vi "Read_Status.vi"(8 "error in (no error)":errorcluster, 11 "Modbus master in":refnum<class "Modbus Master.lvclass">) -> (0 "error out":errorcluster, 2 "Variables":u16[](array[numeric]), 3 "Modbus master out":refnum<class "Modbus Master.lvclass">)   [LabVIEW 2019]
uses:
  <vilib>/Modbus/master/Modbus Master.lvclass
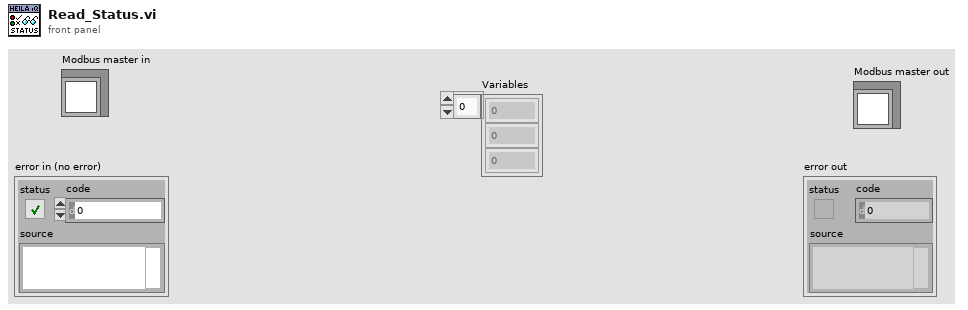
[diagram p1: front panel]
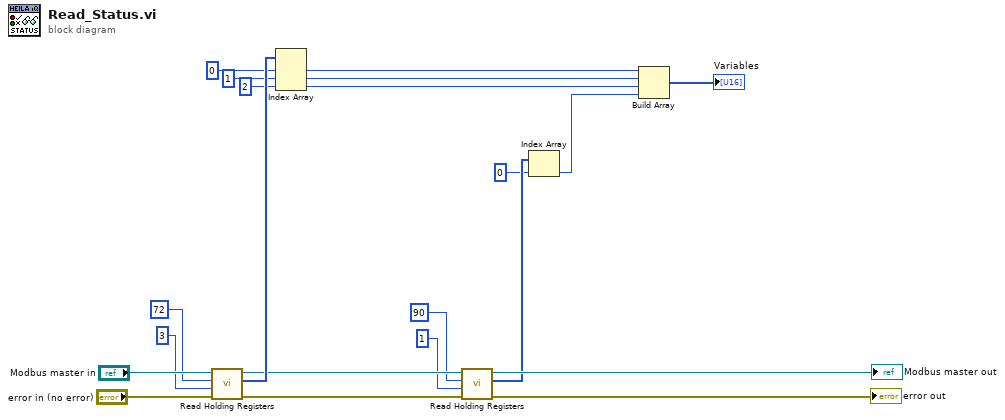
[diagram p0: block diagram]
diagram:
  n1 = call-dynamic "Read Holding Registers.vi"("error in (no error)"="error in (no error)", "number of holding registers"=u16 3 ("starting address"), "starting address"=u16 72, "Modbus master in"="Modbus master in") -> ("error out"=w8:errorcluster, "register values"=w17:u16[], "Modbus master out"=w9:refnum<class "Modbus Master.lvclass">)  [unwired: 5 in]
  n2 = Index Array(array=w17, index #1=0 ("index"), index #2=1 ("index"), index #3=2 ("index")) -> (element #1=w13:u16, element #2=w12:u16, element #3=w11:u16)
  n3 = call-dynamic "Read Holding Registers.vi"("error in (no error)"=w8, "number of holding registers"=u16 1 ("starting address"), "starting address"=u16 90, "Modbus master in"=w9) -> ("error out"=→"error out":errorcluster, "register values"=w3:u16[], "Modbus master out"=→"Modbus master out":refnum<class "Modbus Master.lvclass">)  [unwired: 5 in]
  n4 = Index Array(array=w3, index=0) -> (element=w1:u16)
  n5 = Build Array(w13, w12, w11, w1) -> (→"Variables":u16[])
